vi "find particles (intersecting boundingbox).vi"(1 "Particle Measurements in (bounding boxes)":dbl[][](array[numeric]), 2 "bounding box in":dbl[](array[numeric])) -> (0 "Particles within bounding box":dbl[][](array[numeric]))   [LabVIEW 2013]
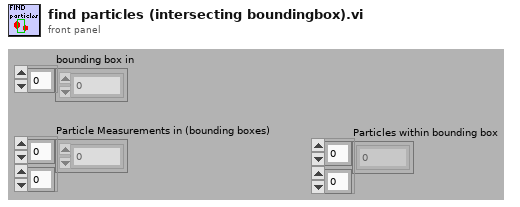
[diagram p1: front panel]
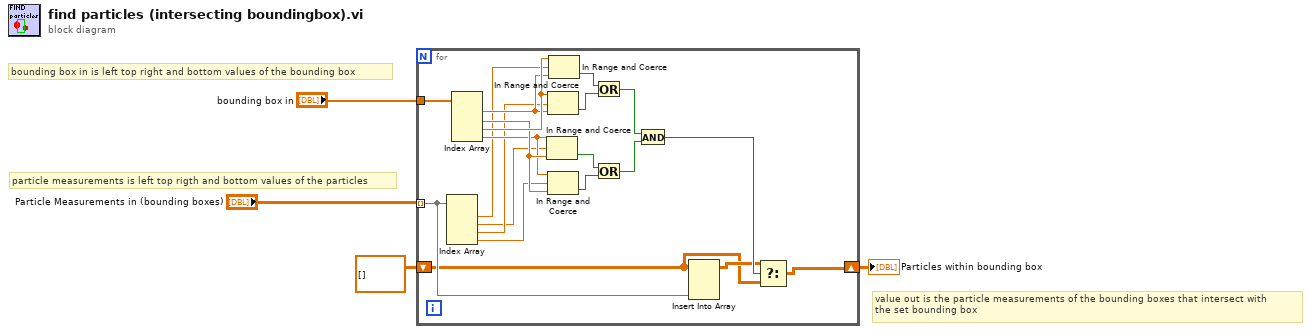
[diagram p0: block diagram]
diagram:
  # "value out is the particle measurements of the bounding boxes that intersect with \nthe set bounding box"
  # "particle measurements is left top rigth and bottom values of the particles"
  # "bounding box in is left top right and bottom values of the bounding box"
  n1 = for {
    tunnel: "bounding box in" -> [w24]
    tunnel: "Particle Measurements in (bounding boxes)" -> [w9] mode=indexing
    shift-right: [w5] -> w1
    shift-left: dbl[][] [] ("array") -> [w6]
    n2 = Index Array(array=w9) -> (element #1=w19:dbl, element #2=w17:dbl, element #3=w18:dbl, element #4=w16:dbl)  [unwired: 4 in]
    n3 = Index Array(array=w24) -> (element #1=w22:dbl, element #2=w21:dbl, element #3=w23:dbl, element #4=w20:dbl)  [unwired: 4 in]
    n4 = In Range and Coerce(upper limit=w20, x=w17, lower limit=w21) -> (In Range?=w14:bool)  [unwired: 1 out]
    n5 = In Range and Coerce(upper limit=w23, x=w18, lower limit=w22) -> (In Range?=w13:bool)  [unwired: 1 out]
    n6 = In Range and Coerce(upper limit=w20, x=w16, lower limit=w21) -> (In Range?=w15:bool)  [unwired: 1 out]
    n7 = In Range and Coerce(upper limit=w23, x=w19, lower limit=w22) -> (In Range?=w12:bool)  [unwired: 1 out]
    n8 = Or(x=w12, y=w13) -> (x .or. y?=w11:bool)
    n9 = Or(x=w14, y=w15) -> (x .or. y?=w10:bool)
    n10 = And(x=w11, y=w10) -> (x .and. y?=w8:bool)
    n11 = Insert Into Array(array=w6, new element=w9) -> (w7:dbl[][])  [unwired: 2 in]
    n12 = Select(t=w7, s=w8, f=w6) -> (s? t:f=w5:dbl[][])
  }
  "Particles within bounding box" <- w1
